vi "Write DUT Info.vi"(8 "error in (no error)":errorcluster, 10 "DUT Info":T1, 11 "Report Information in":refnum<class "Report Information.lvclass">) -> (0 "error out":errorcluster, 3 "Report Information out":refnum<class "Report Information.lvclass">)   [LabVIEW 2015, in "Report Information.lvclass"]
uses:
  Report Information.lvclass
  DUT Information.ctl
  Report Information.lvclass/Report Information.ctl
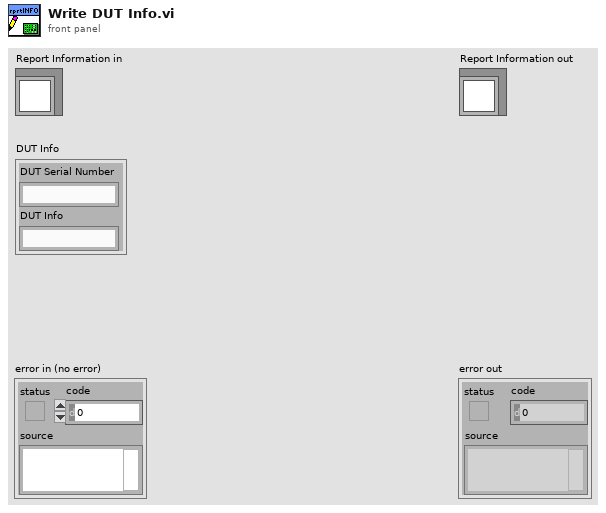
[diagram p1: front panel]
types:
  T1 = typedef "Report Information.lvclass/DUT Information.ctl" = cluster{"DUT Serial Number":string, "DUT Info":string}
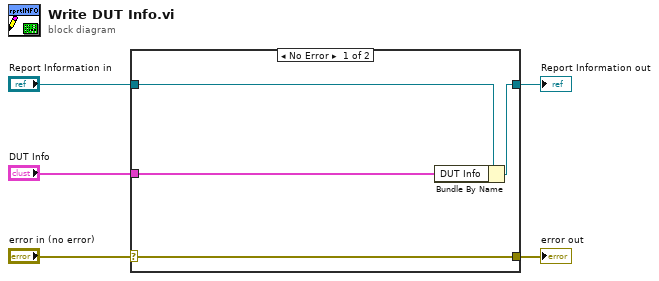
[diagram p0: block diagram]
diagram:
  n1 = case shown="No Error" "error in (no error)" {
    selector: "error in (no error)" -> [w9 w10]
    tunnel: [w9 w10] -> w4
    tunnel: [w7 w11] -> w2
    tunnel: "Report Information in" -> [w8 w11]
    tunnel: "DUT Info" -> [w6 _]
    frame No Error {
      n2 = Bundle By Name(cluster=w8, "DUT Info"=w6) -> (w7:refnum<class "Report Information.lvclass">)
    }
    frame Error {
    }
  }
  "error out" <- w4
  "Report Information out" <- w2
